vi "OAT Get Gap Reference (N Channels).vi"(0 "scaled signals [EU]":waveform(dbl)[](array[waveform]), 2 "reset? (F)":bool, 7 "averaging type":enum16{"Linear", "Exponential"}(ring), 9 "window":T1(ring), 11 "error in (no error)":errorcluster) -> (4 "gap references [V]":dbl[](array[numeric]), 15 "error out":errorcluster)   [LabVIEW 2017, in "SoundVib_RefDataProcess.lvlib"]
doc: "Computes the gap reference of the scaled signal you acquire from a DC-coupled displacement transducer channel. You can subtract the gap reference value from a signal to calculate the actual movement that the displacement transducer measures. Wire data to the <B>scaled signal [EU]</B> input to determine the polymorphic instance to use or manually select the instance."
uses:
  <vilib>/addons/Sound and Vibration/Order Analysis/Referece Data Processing/SoundVib_RefDataProcess.lvlib
  <vilib>/addons/_NISVFA/_Shared subVIs/Common/svc_Check for Waveform Parameter Continuity (no state).vi
  <vilib>/addons/_NISVFA/_Shared subVIs/Common/svc_Engineering Units to Unit Label.vi
  <vilib>/addons/_NISVFA/_Shared subVIs/Common/svc_Unit Label to Engineering Units.vi
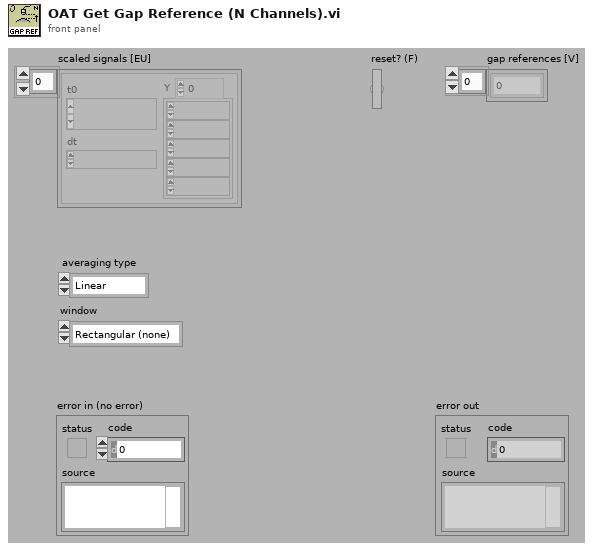
[diagram p1: front panel]
types:
  T1 = enum16{"Rectangular (none)", "Hanning", "Low side lobe"}
  T2 = cluster{"dt equal":bool, "array length equal":bool, "number channels change":bool}
  T3 = cluster{"dt":bool, "t0 continuity":bool, "array length":bool, "channel info":bool, "name":bool}
  T4 = typedef "svc_Channel Info.ctl" = cluster{"sensor sensitivity":dbl, "engineering units":T5, "dB reference":dbl, "custom label":string, "weighting filter":T6, "pregain":dbl}
  T5 = typedef "svc_Engineering Units Text Ring.ctl" = u16
  T6 = typedef "svc_Weighting Filter Text Ring.ctl" = u16
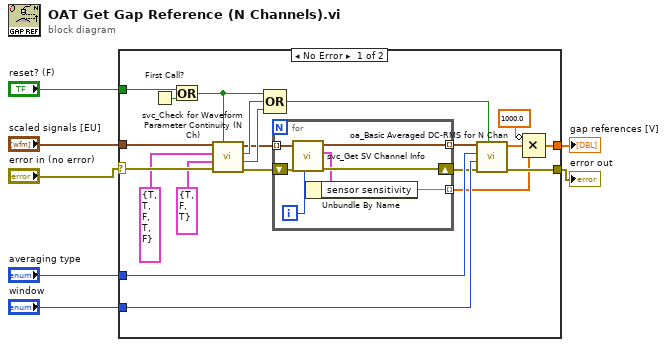
[diagram p0: block diagram]
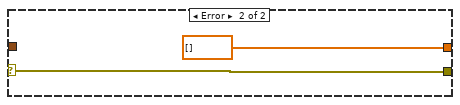
[diagram p2: hidden frame]
diagram:
  n1 = case shown="No Error" "error in (no error)" {
    selector: "error in (no error)" -> [w10 w37]
    tunnel: [w25 w37] -> w2
    tunnel: "scaled signals [EU]" -> [w11 _]
    tunnel: "averaging type" -> [w28 _]
    tunnel: "window" -> [w27 _]
    tunnel: "reset? (F)" -> [w24 _]
    tunnel: [w26 dbl[] []] -> w1
    frame No Error {
      n2 = First Call?() -> (First Call?: T/F=w23:bool)
      n3 = Or(x=w24, y=w23) -> (x .or. y?=w22:bool)
      n4 = call <vilib>:"svc_Check for Waveform Parameter Continuity (N Ch).vi"("restart averaging (F)"=w22, "error in (no error)"=w10, "checks for multichannel parameters"=T2 {"dt equal"=TRUE, "array length equal"=FALSE, "number channels change"=TRUE}, "checks for channel parameter change"=T3 {"dt"=TRUE, "t0 continuity"=TRUE, "array length"=FALSE, "channel info"=TRUE, "name"=FALSE}, "scaled signal(s)"=w11) -> ("error out"=w17:errorcluster, "multichannel parameter changed"=w20:bool, "waveform parameter changed"=w21:bool, "dup scaled signal(s)"=w18:waveform(dbl)[])  [unwired: 3 out]
      n5 = Compound Arithmetic op=OR(w22, w21, w20) -> (w19:bool)
      n6 = for {
        tunnel: w18 -> [w35] mode=indexing
        shift-right: [w33] -> w16
        shift-left: w17 -> [w34]
        tunnel: [w32] -> w15 mode=indexing
        tunnel: [w30] -> w13 mode=indexing
        i -> [w29]
        n7 = call <vilib>:"svc_Get SV Channel Info.vi"("channel index"=w29, "error in (no error)"=w34, "scaled signal [EU]"=w35) -> ("error out"=w33:errorcluster, "channel info"=w31:T4, "dup scaled signal [EU]"=w32:waveform(dbl))  [unwired: 3 in, 3 out]
        n8 = Unbundle By Name(w31) -> ("sensor sensitivity"=w30:dbl)
      }
      n9 = call <vilib>:"oa_Basic Averaged DC-RMS for N Chan.vi"("reset"=w19, "error in (no error)"=w16, "window"=w27, "averaging type"=w28, "signals in"=w15) -> ("error out"=w25:errorcluster, "DC values"=w14:dbl[])  [unwired: 3 in, 2 out]
      n10 = Compound Arithmetic op=MULTIPLY(invert 1000.0 ("sensor sensitivity [mV/EU]"), w14, w13) -> (w26:dbl[])
    }
    frame Error {
    }
  }
  "error out" <- w2
  "gap references [V]" <- w1
